vi "Find Embedded Data Logger Custom Device by Name.vi"(8 "error in":errorcluster, 10 "name":string, 11 "target in":refnum<k39>) -> (0 "error out":errorcluster, 2 "embedded data logger":T1=18446744073709551615 format="%.0x", 3 "target out":refnum<k39>)   [LabVIEW 2027, in "Embedded Data Logger Scripting.lvlib"]
uses:
  Embedded Data Logger Scripting.lvlib
  C:/NetCore/niveristand-embedded-data-logger-custom-device/Source/Scripting/Custom Device/Find Embedded Data Logger Custom Device by Name.vi/NationalInstruments.VeriStand.SystemDefinitionAPI
  NationalInstruments.VeriStand.SystemDefinitionAPI
  <vilib>/NI VeriStand/Custom Device API/Custom Device Item Ref.ctl
  <vilib>/NI VeriStand/Custom Device API/Custom Device API.lvlib
  Shared/Constants.vi
  Shared/Embedded Data Logger Shared.lvlib
  C:/NetCoreDLL/NationalInstruments.VeriStand.SystemDefinitionAPI.dll
  NetCoreDLL/NationalInstruments.VeriStand.SystemDefinitionAPI.dll
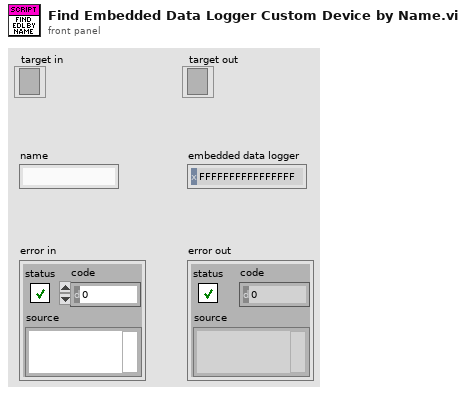
[diagram p1: front panel]
types:
  T1 = typedef "Custom Device API.lvlib/Custom Device Item Ref.ctl" = u64
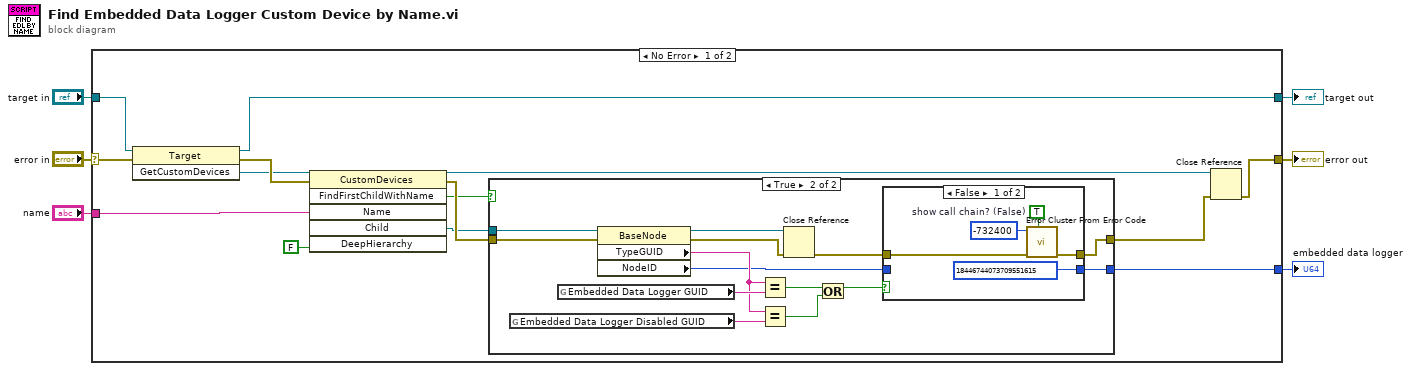
[diagram p0: block diagram]
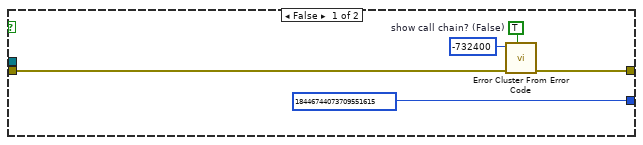
[diagram p2: hidden frame]
diagram:
  n1 = case shown="No Error" "error in" {
    selector: "error in" -> [w17 w47]
    tunnel: "target in" -> [w18 w48]
    tunnel: [w15 w48] -> w4
    tunnel: [w12 w47] -> w3
    tunnel: [w9 _] -> w1
    tunnel: "name" -> [w10 _]
    frame No Error {
      n2 = invoke class="Target" method="GetCustomDevices"(reference=w18, error in=w17) -> (reference out=w15:refnum<k39>, error out=w20:errorcluster, "GetCustomDevices"=w19:refnum<k39>)  [unwired: 1 in]
      n3 = invoke class="CustomDevices" method="FindFirstChildWithName"(reference=w19, error in=w20, "Name"=w10, "DeepHierarchy"=FALSE) -> (reference out=w13:refnum<k39>, error out=w16:errorcluster, "FindFirstChildWithName"=w7:bool, "Child"=w8:refnum<k39>)  [unwired: 2 in, 2 out]
      n4 = case shown="True" w7 {
        tunnel: w16 -> [w21 w39]
        tunnel: [w22 w32] -> w14
        tunnel: [T1 18446744073709551615 ("embedded data logger custom device") w36] -> w9
        tunnel: w8 -> [_ w37]
        frame False {
          w24 = TRUE  # show call chain? (False)
          n5 = call <vilib>:"Error Cluster From Error Code.vi"("show call chain? (False)"=w24, "error in (no error)"=w21, "error code (0)"=-732400) -> ("error out"=w22:errorcluster)  [unwired: 6 in]
        }
        frame True {
          n6 = global read "Constants.vi" "Embedded Data Logger Disabled GUID"() -> (w28:string)
          n7 = global read "Constants.vi" "Embedded Data Logger GUID"() -> (w34:string)
          n8 = property class="BaseNode"(reference=w37, error in=w39) -> (reference out=w38:refnum<k39>, error out=w35:errorcluster, "TypeGUID"=w27:string, "NodeID"=w26:u64)
          n9 = Equal?(x=w27, y=w34) -> (x = y?=w31:bool)
          n10 = Equal?(x=w27, y=w28) -> (x = y?=w29:bool)
          n11 = Close Reference(reference=w38, error in (no error)=w35) -> (error out=w33:errorcluster)
          n12 = Or(x=w31, y=w29) -> (x .or. y?=w30:bool)
          n13 = case shown="False" w30 {
            tunnel: w26 -> [_ w46]
            tunnel: [T1 18446744073709551615 ("embedded data logger custom device") w46] -> w36
            tunnel: w33 -> [w43 w45]
            tunnel: [w42 w45] -> w32
            frame False {
              w41 = TRUE  # show call chain? (False)
              n14 = call <vilib>:"Error Cluster From Error Code.vi"("show call chain? (False)"=w41, "error in (no error)"=w43, "error code (0)"=-732400) -> ("error out"=w42:errorcluster)  [unwired: 6 in]
            }
            frame True {
            }
          }
        }
      }
      n15 = Close Reference(reference=w13, error in (no error)=w14) -> (error out=w12:errorcluster)
    }
    frame Error {
    }
  }
  "target out" <- w4
  "error out" <- w3
  "embedded data logger" <- w1
